vi "Synthesize.vi"(0 "Channel in":refnum<class "Channel.lvclass">, 5 "Fs (Hz)":dbl, 7 "Npts":i32, 9 "Repetition":i32, 11 "error in (no error)":errorcluster, 12 "last":bool) -> (4 "Channel out":refnum<class "Channel.lvclass">, 6 "Number":i32, 8 "Array":dbl[](array[numeric]), 15 "error out":errorcluster)   [LabVIEW 2020, in "Channel.lvclass"]
uses:
  Channel.lvclass
  Channel.lvclass/Channel.ctl
  Waveforms/Waveform/Waveform.lvclass
  Modulations/AM/AM.lvclass
  Gate/Gate.lvclass
  Level/Level.lvclass
  Filter/Filter.lvclass
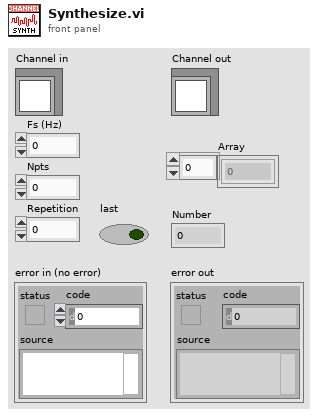
[diagram p1: front panel]
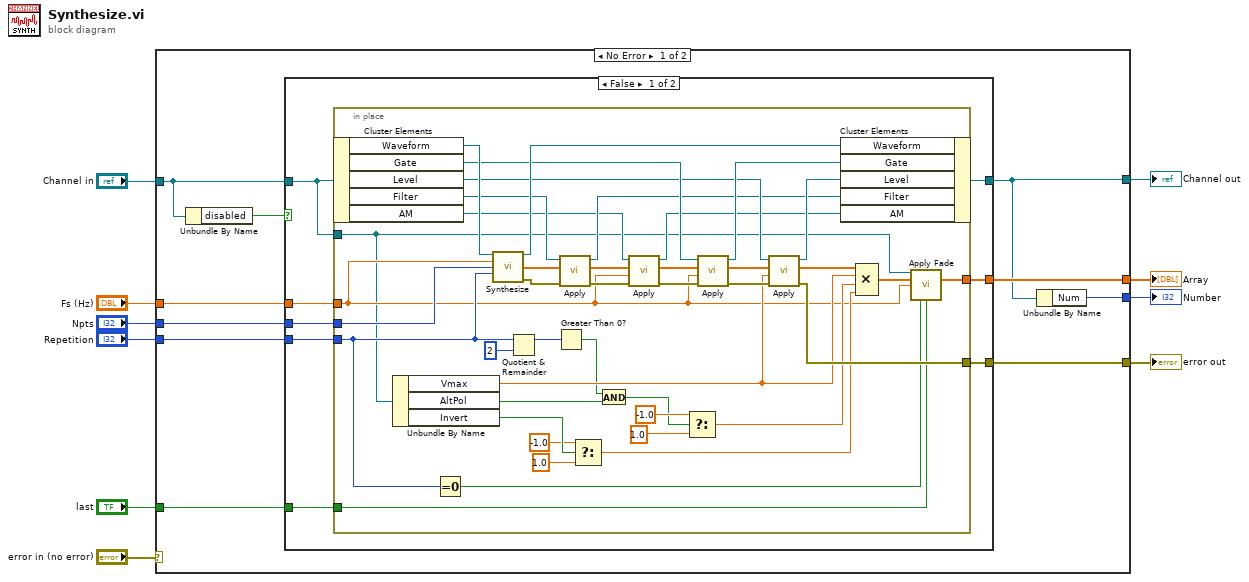
[diagram p0: block diagram]
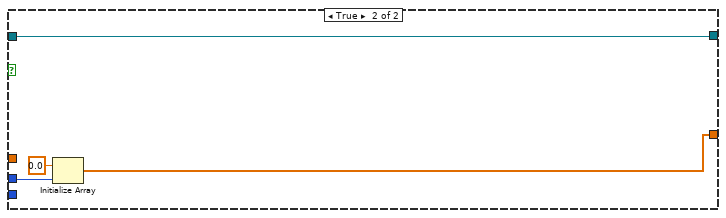
[diagram p2: hidden frame]
diagram:
  n1 = case shown="No Error" "error in (no error)" {
    selector: "error in (no error)" -> [_ w75]
    tunnel: [w14 w75] -> w9
    tunnel: [w16 w74] -> w7
    tunnel: "Channel in" -> [w12 w74]
    tunnel: "Fs (Hz)" -> [w20 _]
    tunnel: "Npts" -> [w19 _]
    tunnel: "Repetition" -> [w18 _]
    tunnel: [w17 _] -> w3
    tunnel: [w15 _] -> w2
    tunnel: "last" -> [w11 _]
    frame No Error {
      n2 = Unbundle By Name(w12) -> ("disabled"=w13:bool)
      n3 = case shown="False" w13 {
        tunnel: w20 -> [w28 _]
        tunnel: w19 -> [w27 w73]
        tunnel: w18 -> [w26 _]
        tunnel: [w25 w71] -> w17
        tunnel: [w24 w70] -> w16
        tunnel: [w23 _] -> w14
        tunnel: w12 -> [w22 w70]
        tunnel: w11 -> [w21 _]
        frame False {
          n4 = in-place {
            in-place-border: w28 -> [w33]
            in-place-border: w27 -> [w68]
            in-place-border: w26 -> [w34]
            in-place-border: [w32] -> w25
            in-place-border: [w59] -> w23
            in-place-border: w22 -> [w31]
            in-place-border: w21 -> [w29]
            n5 = in-place-cluster #1(w22) -> ("Waveform"=w69:refnum<class "Waveform.lvclass">, "Gate"=w66:refnum<class "Gate.lvclass">, "Level"=w63:refnum<class "Level.lvclass">, "Filter"=w56:refnum<class "Filter.lvclass">, "AM"=w49:refnum<class "AM.lvclass">)
            n6 = Unbundle By Name(w31) -> ("Vmax"=w54:dbl, "AltPol"=w41:bool, "Invert"=w47:bool)
            n7 = Equal To 0?(x=w34) -> (x = 0?=w30:bool)
            n8 = call-dynamic "Synthesize.vi"("Waveform in"=w69, "Fs (Hz)"=w33, "Npts"=w68, "Repetition"=w34) -> ("Waveform out"=w67:refnum<class "Waveform.lvclass">, "Array"=w58:dbl[], "error out"=w57:errorcluster)  [unwired: 9 in]
            n9 = Quotient & Remainder(x=w34, y=2) -> (x-y*floor(x/y)=w43:i32)  [unwired: 1 out]
            n10 = Greater Than 0?(x=w43) -> (x > 0?=w40:bool)
            n11 = call "Apply.vi"("error in (no error)"=w57, "Array in"=w58, "Filter in"=w56) -> ("error out"=w50:errorcluster, "Array out"=w53:dbl[], "Filter out"=w55:refnum<class "Filter.lvclass">)  [unwired: 6 in]
            n12 = Select(t=-1.0, s=w47, f=1.0) -> (s? t:f=w36:dbl)
            n13 = And(x=w40, y=w41) -> (x .and. y?=w39:bool)
            n14 = call-dynamic "Apply.vi"("error in (no error)"=w50, "Fs (Hz)"=w33, "Array in"=w53, "AM in"=w49) -> ("error out"=w51:errorcluster, "Array out"=w52:dbl[], "AM out"=w48:refnum<class "AM.lvclass">)  [unwired: 5 in]
            n15 = Select(t=-1.0, s=w39, f=1.0) -> (s? t:f=w37:dbl)
            n16 = call "Apply.vi"("error in (no error)"=w51, "Fs (Hz)"=w33, "Array in"=w52, "Gate in"=w66) -> ("error out"=w60:errorcluster, "Array out"=w64:dbl[], "Gate out"=w65:refnum<class "Gate.lvclass">)  [unwired: 5 in]
            n17 = call "Apply.vi"("error in (no error)"=w60, "Vmax"=w54, "Array in"=w64, "Level in"=w63) -> ("error out"=w59:errorcluster, "Array out"=w61:dbl[], "Level out"=w62:refnum<class "Level.lvclass">)  [unwired: 5 in]
            n18 = in-place-cluster #1("Waveform"=w67, "Gate"=w65, "Level"=w62, "Filter"=w55, "AM"=w48) -> (w24:refnum<class "Channel.lvclass">)
            n19 = Compound Arithmetic op=MULTIPLY(w61, w54, w37, w36) -> (w35:dbl[])
            n20 = call "Apply Fade.vi"("Channel in"=w31, "Array in"=w35, "Fs (Hz)"=w33, "first"=w30, "last"=w29) -> ("Array out"=w32:dbl[])  [unwired: 8 in, 2 out]
          }
        }
        frame True {
          n21 = Initialize Array(0.0, w73) -> (w71:dbl[])
        }
      }
      n22 = Unbundle By Name(w16) -> ("Num"=w15:i32)
    }
    frame Error {
    }
  }
  "error out" <- w9
  "Channel out" <- w7
  "Number" <- w2
  "Array" <- w3
